vi "Framework Simulation.vi"() -> ()   [LabVIEW 2016]
uses:
  Simulated DSF Custom Device/Simulated DSF Custom Device.lvclass
  C:/Git/SourceTree/DSF/Development/Testing/Simulated VeriStand Custom Device/Simulated VeriStand Custom Device.lvclass
  Simulated VeriStand Custom Device/Simulated VeriStand Custom Device.lvclass
  Source/Submodules/Memory/Source/Classes/Pointer/Memory.Pointer.lvclass/Memory.Pointer.ctl
  Simulated VeriStand Engine/Accessors/Set Channel Count.vi
  Source/Submodules/Memory/Source/Classes/Internal/Memory.Pointer.Internal.New.vi
  Simulated VeriStand Engine/Accessors/Write Control Pointers.vi
  Simulated VeriStand Engine/Accessors/Write Status Pointers.vi
  Source/Submodules/Memory/Source/Classes/Pointer/Memory.Pointer.Write.vi
  Source/Submodules/Memory/Source/Classes/Pointer/Memory.Pointer.Write.Safe.0D.Bool.vi
  Source/Submodules/Memory/Source/Classes/Pointer/Memory.Pointer.Write.Safe.0D.U32.vi
  Simulated VeriStand Engine/Accessors/Write Data Ref.vi
  Source/Submodules/Memory/Source/Classes/Pointer/Memory.Pointer.Write.Unsafe.0D.Bool.vi
  Source/Submodules/Memory/Source/Classes/Pointer/Memory.Pointer.Parameter Check.Null Pointer.vi
  Source/Submodules/Memory/Source/Classes/Pointer/Memory.Pointer.Parameter Check.Subset.vi
  Source/Submodules/Memory/Source/Classes/Pointer/Memory.Pointer.Write.Unsafe.0D.U32.vi
  Source/Submodules/Memory/Source/Classes/Pointer/Memory.Pointer.Get Address.vi
  Source/Submodules/Memory/Source/Classes/Pointer/Memory.Pointer.Errors.vi
  Source/Submodules/Memory/Source/Classes/Pointer/Memory.Pointer.Errors.Null Pointer.vi
  Source/Submodules/Memory/Source/Classes/Pointer/Memory.Pointer.Errors.Out of Bounds.vi
  Source/Submodules/Memory/Source/Classes/Pointer/Memory.Pointer.Get Size.vi
  Source/Submodules/Memory/Source/Classes/Pointer/Memory.Pointer.Errors.Create Error.vi
  Source/Submodules/Memory/Source/Submodules/SEH/Source/VIs/Static Error Handling.Source Buffer.Write.String.vi
  Source/Submodules/Memory/Source/Classes/Pointer/Memory.Pointer.Errors.Write Pointer Size.vi
  Source/Submodules/Memory/Source/Submodules/SEH/Source/VIs/Static Error Handling.Source Buffer.Write.Numeric.Scalar.Base10.vi
  Source/Submodules/Memory/Source/Submodules/SEH/Source/VIs/Static Error Handling.Source Buffer.Write.Numeric.Scalar.Base10 (U64).vi
  Source/Submodules/Memory/Source/Submodules/SEH/Source/VIs/Static Error Handling.Error Cluster Constant.vi
  Source/Submodules/Memory/Source/Submodules/SEH/Source/VIs/Static Error Handling.Error Cluster Constant (256B).vi
  Source/Submodules/Memory/Source/Submodules/SEH/Source/VIs/Static Error Handling.Parameters.Status.Set.vi
  Source/Submodules/Memory/Source/Submodules/SEH/Source/VIs/Static Error Handling.Parameters.Code.Set.vi
  Source/Submodules/Memory/Source/Submodules/SEH/Source/VIs/Static Error Handling.Parameters.VI Source.Set.vi
  Source/Submodules/Memory/Source/Constants/Memory.Constants.vi
  Source/Submodules/Memory/Source/Constants/Memory.Constants.Library Name.vi
  Source/Submodules/Memory/Source/Classes/Pointer/Memory.Pointer.Errors.Get Info.vi
  Source/Submodules/Memory/Source/Classes/Internal/Memory.Pointer.Internal.lvclass
  C:/Git/SourceTree/DSF/Source/Submodules/Memory/Source/Classes/Pointer/Memory.Pointer.lvclass
  <vilib>/NI Veristand/Custom Device API/Global Data Refs.vi
  Source/Submodules/Memory/Source/Classes/Internal/Memory.Pointer.Internal.Allocate.vi
  Simulated VeriStand Engine/Simulated VeriStand Engine.lvclass
panel:
  in  "Channel Count":u32
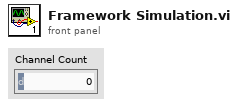
[diagram p1: front panel]
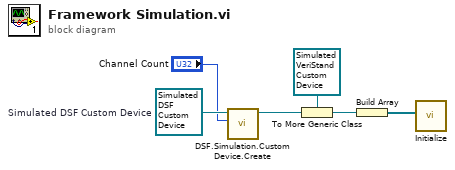
[diagram p0: block diagram]
diagram:
  w5 = refnum<class "Simulated DSF Custom Device.lvclass"> refnum  # Simulated DSF Custom Device
  n1 = call "DSF.Simulation.Custom Device.Create.vi"("Channel Count"="Channel Count", "Simulated VeriStand Custom Device in"=w5) -> ("Simulated VeriStand Custom Device out"=w4:refnum<class "Simulated DSF Custom Device.lvclass">)  [unwired: 8 in, 1 out]
  n2 = To More Generic Class(target class=refnum<class "Simulated VeriStand Custom Device.lvclass"> refnum ("Simulated VeriStand Custom Device out"), reference=w4) -> (generic class reference=w2:refnum<class "Simulated VeriStand Custom Device.lvclass">)
  n3 = Build Array(w2) -> (w6:refnum<class "Simulated VeriStand Custom Device.lvclass">[])
  n4 = call "Initialize.vi"("Simulated Custom Devices"=w6) -> ()  [unwired: 9 in, 2 out]
